vi "Check Optimisation Status.vi"(8 "error in (no error)":errorcluster, 11 "Monkey in":refnum<class "Monkey.lvclass">) -> (0 "error out":errorcluster, 2 "Optimiser":bool, 3 "Monkey out":refnum<class "Monkey.lvclass">)   [LabVIEW 2020, in "TALOS.lvlib" / "Monkey.lvlib" / "Monkey.lvclass"]
doc: "VI checks if the next active cell is an optimisation cell"
uses:
  Monkey.lvclass
  Monkey.lvclass/Monkey.ctl
  Run Utilities/Run Block/Run Block.lvclass
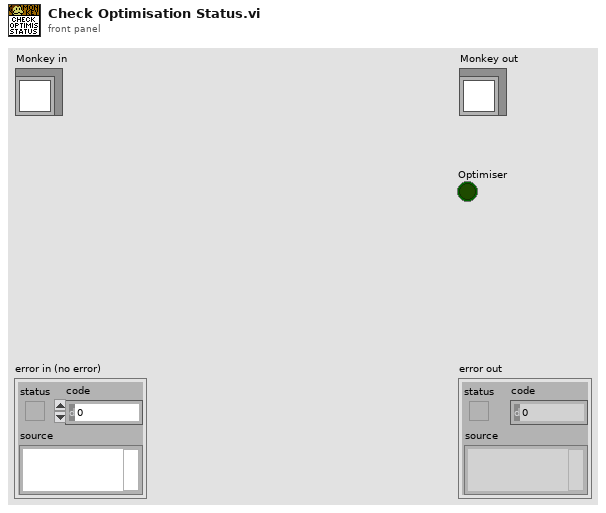
[diagram p1: front panel]
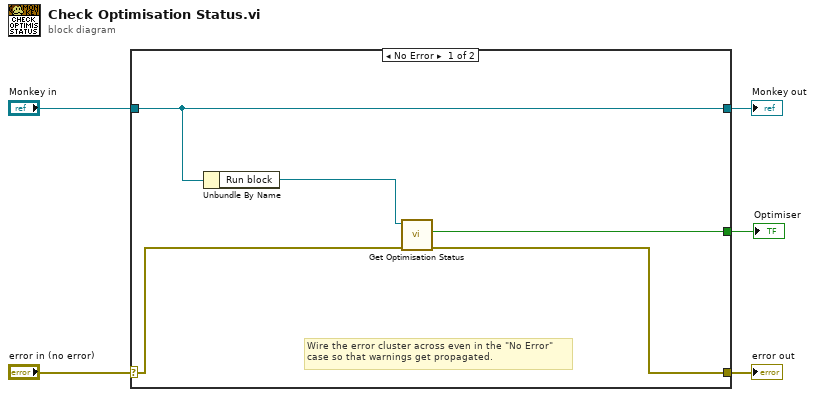
[diagram p0: block diagram]
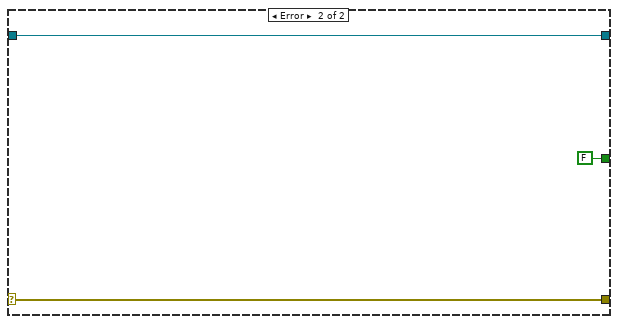
[diagram p2: hidden frame]
diagram:
  n1 = case shown="No Error" "error in (no error)" {
    selector: "error in (no error)" -> [w9 w13]
    tunnel: [w8 w13] -> w4
    tunnel: [w10 w12] -> w2
    tunnel: "Monkey in" -> [w10 w12]
    tunnel: [w6 FALSE ("Optimiser")] -> w1
    frame No Error {
      # "Wire the error cluster across even in the \"No Error\"\ncase so that warnings get propagated."
      n2 = Unbundle By Name(w10) -> ("Run block"=w7:refnum<class "Run Block.lvclass">)
      n3 = call-dynamic "Get Optimisation Status.vi"("error in (no error)"=w9, "Run Block in"=w7) -> ("error out"=w8:errorcluster, "Optimiser"=w6:bool)  [unwired: 7 in, 1 out]
    }
    frame Error {
    }
  }
  "error out" <- w4
  "Monkey out" <- w2
  "Optimiser" <- w1
